vi "emi_Read System ID.vi"(9 "error in (no error)":errorcluster) -> (8 "System ID":u8, 10 "error out":errorcluster)   [LabVIEW 2011]
doc: "Checks wheter the application id closeing,"
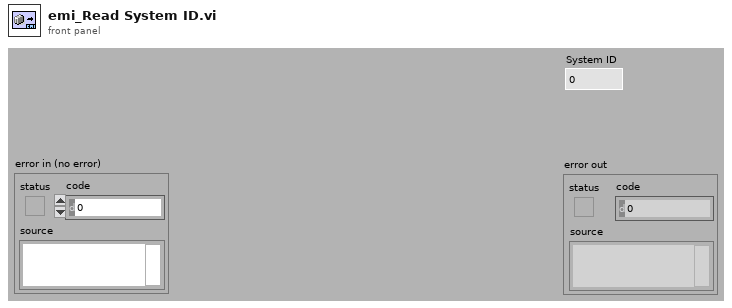
[diagram p1: front panel]
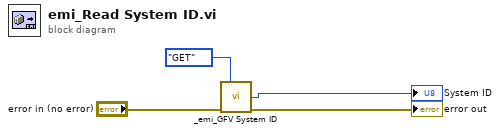
[diagram p0: block diagram]
diagram:
  n1 = call "_emi_GFV System ID.vi"("Action(GET)"=enum16{"GET", "SET"}."GET", "error in (no error)"="error in (no error)") -> ("System ID out"=→"System ID":u8, "error out"=→"error out":errorcluster)  [unwired: 12 in]
